vi "ke37xx Get Calibration Date.vi"(8 "error in (no error)":errorcluster, 10 "Card Slot":u8=1 min=1 max=6 step=1, 11 "VISA Resource Name":refnum<visa-resource-name>) -> (0 "error out":errorcluster, 1 "Date Card Calibrated":string, 3 "VISA Resource Name Out":refnum<visa-resource-name>)   [LabVIEW 2009, in "Keithley 3700 Series.lvlib"]
doc: "This VI returns the date the card was last calibrated in MM/DD/YYYY format."
uses:
  <instrlib>/Keithley 3706/Keithley 3700 Series.lvlib
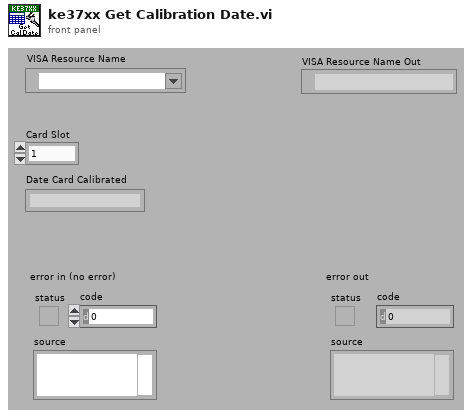
[diagram p1: front panel]
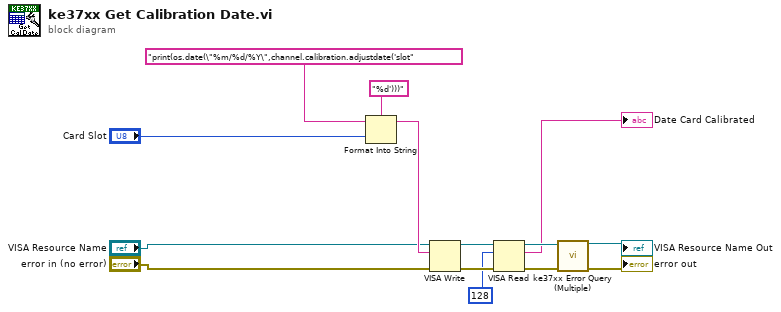
[diagram p0: block diagram]
diagram:
  n1 = Format Into String(format string="%d')))", initial string="print(os.date(\"%m/%d/%Y\",channel.calibration.adjustdate('slot", "Card Slot") -> (resulting string=w12:string)  [unwired: 1 in, 1 out]
  n2 = VISA Write(VISA resource name="VISA Resource Name", write buffer=w12, error in (no error)="error in (no error)") -> (VISA resource name out=w7:refnum<visa-resource-name>, error out=w6:errorcluster)  [unwired: 1 out]
  n3 = VISA Read(VISA resource name=w7, byte count=128, error in (no error)=w6) -> (VISA resource name out=w8:refnum<visa-resource-name>, read buffer=→"Date Card Calibrated":string, error out=w9:errorcluster)  [unwired: 1 out]
  n4 = call <instrlib>:"ke37xx Error Query (Multiple).vi"("VISA resource name"=w8, "error in (no error)"=w9) -> ("VISA resource name out"=→"VISA Resource Name Out":refnum<visa-resource-name>, "error out"=→"error out":errorcluster)  [unwired: 12 out]
